vi "Read configuration.vi"(7 "force loading?":bool=TRUE, 8 "error in (no error)":errorcluster, 11 "ServiceManager in":refnum<class "ServiceManager.lvclass">) -> (0 "error out":errorcluster, 3 "ServiceManager out":refnum<class "ServiceManager.lvclass">)   [LabVIEW 2012, in "ServiceManager.lvclass"]
uses:
  ServiceManager.lvclass
  Murmex/LabVIEW/Murmex/Murmex/Murmex.lvclass
  ServiceManager.lvclass/ServiceManager.ctl
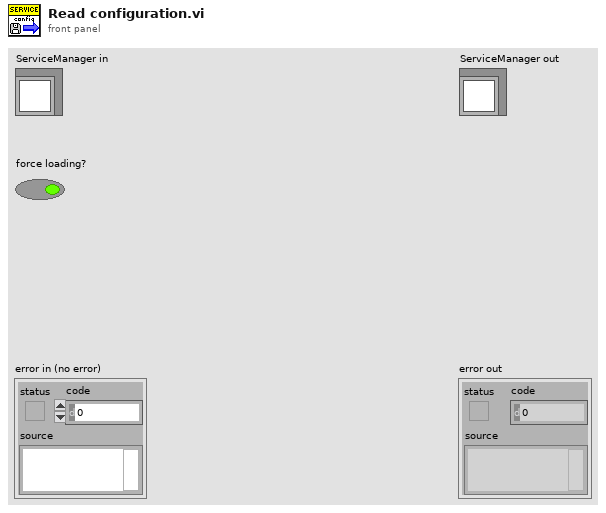
[diagram p1: front panel]
types:
  T1 = typedef "ServiceManager.lvclass/configuration_cluster.ctl" = cluster{"search paths":string[]}
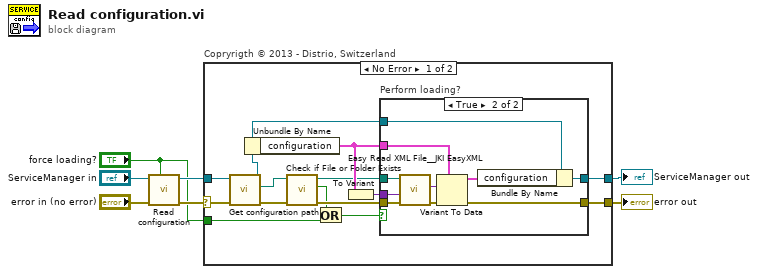
[diagram p0: block diagram]
diagram:
  n1 = call-parent "Read configuration.vi"("force loading?"="force loading?", "error in (no error)"="error in (no error)", "Murmex in"="ServiceManager in") -> ("error out"=w5:errorcluster, "Murmex out"=w4:refnum<class "ServiceManager.lvclass">)  [unwired: 7 in]
  n2 = case "Copryrigth © 2013 - Distrio, Switzerland" shown="No Error" w5 {
    selector: w5 -> [w12 w35]
    tunnel: [w18 w35] -> w1
    tunnel: [w21 w34] -> w2
    tunnel: w4 -> [w9 w34]
    tunnel: "force loading?" -> [w17 _]
    frame No Error {
      n3 = call "Get configuration path.vi"("error in (no error)"=w12, "Murmex in"=w9) -> ("error out"=w11:errorcluster, "configuration path"=w10:path, "Murmex out"=w8:refnum<class "ServiceManager.lvclass">)  [unwired: 7 in]
      n4 = Unbundle By Name(w8) -> ("configuration"=w19:T1)
      n5 = call <vilib>:"Check if File or Folder Exists.vi"("error in (no error)"=w11, "path"=w10) -> ("error out"=w14:errorcluster, "file or folder exists?"=w13:bool, "dup path"=w15:path)  [unwired: 7 in]
      n6 = Or(x=w13, y=w17) -> (x .or. y?=w16:bool)
      n7 = To Variant(anything=w19) -> (Variant=w20:variant)
      n8 = case "Perform loading?" shown="True" w16 {
        tunnel: [w23 w25] -> w21
        tunnel: w20 -> [_ w32]
        tunnel: w19 -> [_ w31]
        tunnel: [w22 w24] -> w18
        tunnel: w15 -> [_ w29]
        tunnel: w14 -> [w22 w28]
        tunnel: w8 -> [w23 w27]
        frame False {
        }
        frame True {
          n9 = call <vilib>:"Easy Read XML File__JKI EasyXML.vi"("error in (no error)"=w28, "LabVIEW Data (Type)"=w32, "XML File Path"=w29) -> ("error out"=w30:errorcluster, "LabVIEW Data"=w33:variant)  [unwired: 6 in, 1 out]
          n10 = Variant To Data(error in=w30, type=w31, Variant=w33) -> (data=w26:T1, error out=w24:errorcluster)
          n11 = Bundle By Name(cluster=w27, "configuration"=w26) -> (w25:refnum<class "ServiceManager.lvclass">)
        }
      }
    }
    frame Error {
    }
  }
  "error out" <- w1
  "ServiceManager out" <- w2
